vi "NML Data Acquisition Setup 1.00.vi"(9 "Parameters Input":T1={"Magnetic Field"=0.0, "Temperature"=0.0, "Exposure Time"=0.0, "Mag ID string"="", "User Name"="Albert Einstein", "Comments"="", "SaveComments?"=1, "X-Axis Unit"=1, "Delimiter"=0, "File Format"=0, "Sample Name"="Sample1"} {"File Format" items=["Macintosh (EOL: CR)", "Unix (EOL: LF)", "DOS/Windows (EOL: CR+LF)"]; "Delimiter" items=["TAB", "COMMA", "SPACE"]; "X-Axis Unit" items=["Point #", "nm", "eV", "meV", "cm-1"]; "SaveComments?" items=["Bare data only", "Saved in the Header Area", "Saved as a Parameter File"]; "Exposure Time" format="%.2f"; "Temperature" format="%.2f"; "Magnetic Field" format="%.2f"}) -> (0 "McP Scan Parameter":T2={"McP on?"=TRUE, "Wait"=0.0, "X-Axis Unit String"="", "Data Format"=0, "Scanning Pattern:"=0, "Spex on?"=TRUE} {"Scanning Pattern:" items=["Uniform Points ", "User Defined Point Pattern ", "Time-Drive"]; "Data Format" items=["Original", "1024rows X 2cloumns", "Future Use"]; "Wait" format="%.2f"}, 3 "Parameters Output":T1={"Magnetic Field"=0.0, "Temperature"=0.0, "Exposure Time"=0.0, "Mag ID string"="", "User Name"="Albert Einstein", "Comments"="", "SaveComments?"=1, "X-Axis Unit"=1, "Delimiter"=0, "File Format"=0, "Sample Name"="Sample1"} {"File Format" items=["Macintosh (EOL: CR)", "Unix (EOL: LF)", "DOS/Windows (EOL: CR+LF)"]; "Delimiter" items=["TAB", "COMMA", "SPACE"]; "X-Axis Unit" items=["Point #", "nm", "eV", "meV", "cm-1"]; "SaveComments?" items=["Bare data only", "Saved in the Header Area", "Saved as a Parameter File"]; "Exposure Time" format="%.2f"; "Temperature" format="%.2f"; "Magnetic Field" format="%.2f"})   [LabVIEW 2024]
doc: "VI which calls the appropriate GPIB routines for a variety of instruments.\nScott Hannahs, NHMFL-FSU, Nov. 1993"
uses:
  Sub Controls/NML GPIB List.ctl
  Sub VIs/McP Parameter.ctl
  xwei previous work/CCD Project/Subroutines/Parameters#1.ctl
  Globals and TypeDefs/Global Varibal Control.vi
panel:
  in  "Data Format":u8(ring)=1 items=["Original", "1024rows X 2cloumns", "Future Use"]
  in  "Spex1680 on?":bool=TRUE caption="Off"
  in  "X-Axis Unit String":string[](array[string])=["nm", "nm", "eV", "meV", "cm_1"]
  out "GPIB Status":string
  in  "ScanPattern":string="1.300000\r1.310000\r1.320000\r1.330000\r1.340000\r1.350000\r1.360000\r1.370000\r1.380000\r1.390000\r1.400000\r"
  in  "Logcluster":T3
  in  "Wait":dbl=1.0 caption="Wait(sec)" min=0.0 max=10000.0 format="%.1f"
  in  "Cancel":bool
  in  "Scanning Pattern:":u32(ring) items=["Uniform Points (Stop-&-Go)", "User Defined Point Pattern (Stop-&-Go)", "Time-Drive (Spectrometer moves at a constant speed)"]
  in  "End Point":dbl=1600.0 min=0.0 max=1000000.0 format="%.3f"
  in  "#Points":u16=100 min=2
  in  "Step":dbl=6.0 min=1e-05 format="%.3f"
  in  "Start Point":dbl=1000.0 min=0.0 max=1000000.0 format="%.3f"
  out "Clock":string="10:27:18 AM"
  in  "McP on?":bool=TRUE caption="Off"
  in  "Done?":bool
  in  "BusScan?":bool
  in  "SaveComments?":u16(ring)=1 items=["Bare data only", "Saved in the Header Area", "Saved as a Parameter File"]
  in  "Delimiter":u16(ring) items=["TAB", "COMMA", "SPACE"]
  in  "File Format":u16(ring) items=["Macintosh (EOL: CR)", "Unix (EOL: LF)", "DOS/Windows (EOL: CR+LF)"]
  in  "User Name":string="Conan The Scientist"
  in  "Sample Name":string="Sample1"
  in  "error in (no error)":errorcluster
  out "error out":errorcluster
  # "Scanning Panel"
  # "User Profile Panel"
  # "GPIB Instruments Panel"
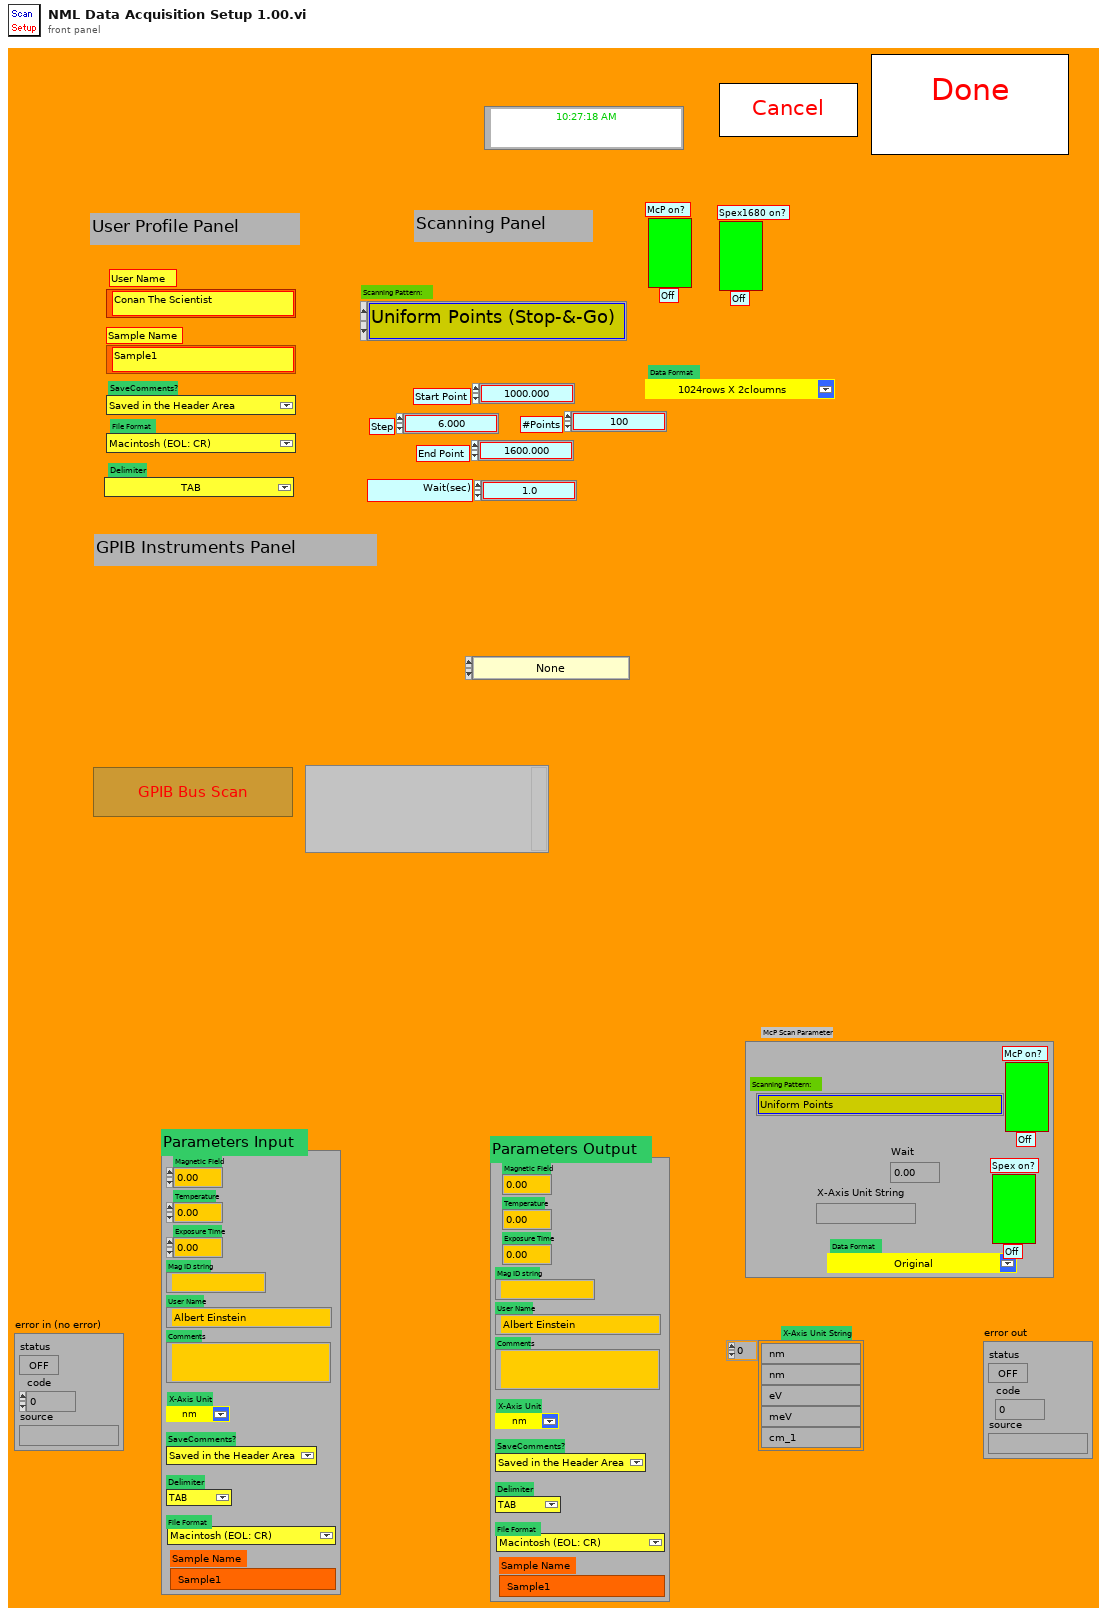
[diagram p1: front panel]
types:
  T1 = typedef "Parameters#1.ctl" = cluster{"Magnetic Field":dbl, "Temperature":dbl, "Exposure Time":dbl, "Mag ID string":string, "User Name":string, "Comments":string, "SaveComments?":u16, "X-Axis Unit":u16, "Delimiter":u16, "File Format":u16, "Sample Name":string}
  T2 = typedef "McP Parameter.ctl" = cluster{"McP on?":bool, "Wait":dbl, "X-Axis Unit String":string, "Data Format":u8, "Scanning Pattern:":u32, "Spex on?":bool}
  T3 = typedef "NML GPIB List.ctl" = enum16{"None", "Field", "Field - SCM1", "DMM", "DMM - HP 34401", "Keithley 2XXX", "Running DMM Ave", "Running HP34401", "Running K2XXX Ave", "SRS 830 - CH 1", "SRS 830 - CH1 & 2", "SRS PTC10", "Signal Rec 7265 - X", "Signal Rec 7265 - X&Y", "DRC 93C - Sample", "DRC 93C - Control", "DRC 93C - Sam&Con", "CryoCon Sensor A", "CryoCon Sensor B", "Cond 20C Sensor 1", "Cond 20C Sensor 2", "LS 336 Read", "LS 340 Read", "LS 370 Read", "LS 370 Select", "AVS 46 Bridge", "BLM Rotator Read Position", "Linear Research 700", "LR 700 Select", "Keithley 3330 - LCZ", "A-H Capacitance", "Digital Integrator", "SRS 400 Phot Ctr", "LakeShore VSM", "AMI He Level Meter", "Time Stamp", "Wait", "Invert Current", "K230 Linear V", "K230 VÅB^2", "Temp Ramp", "Power Ramp", "Freq Sweep", "LTC Stable T", "Scanner Step", "IMS Stepper Increment", "BLM Stepper Increment", "Omega CNi32"}
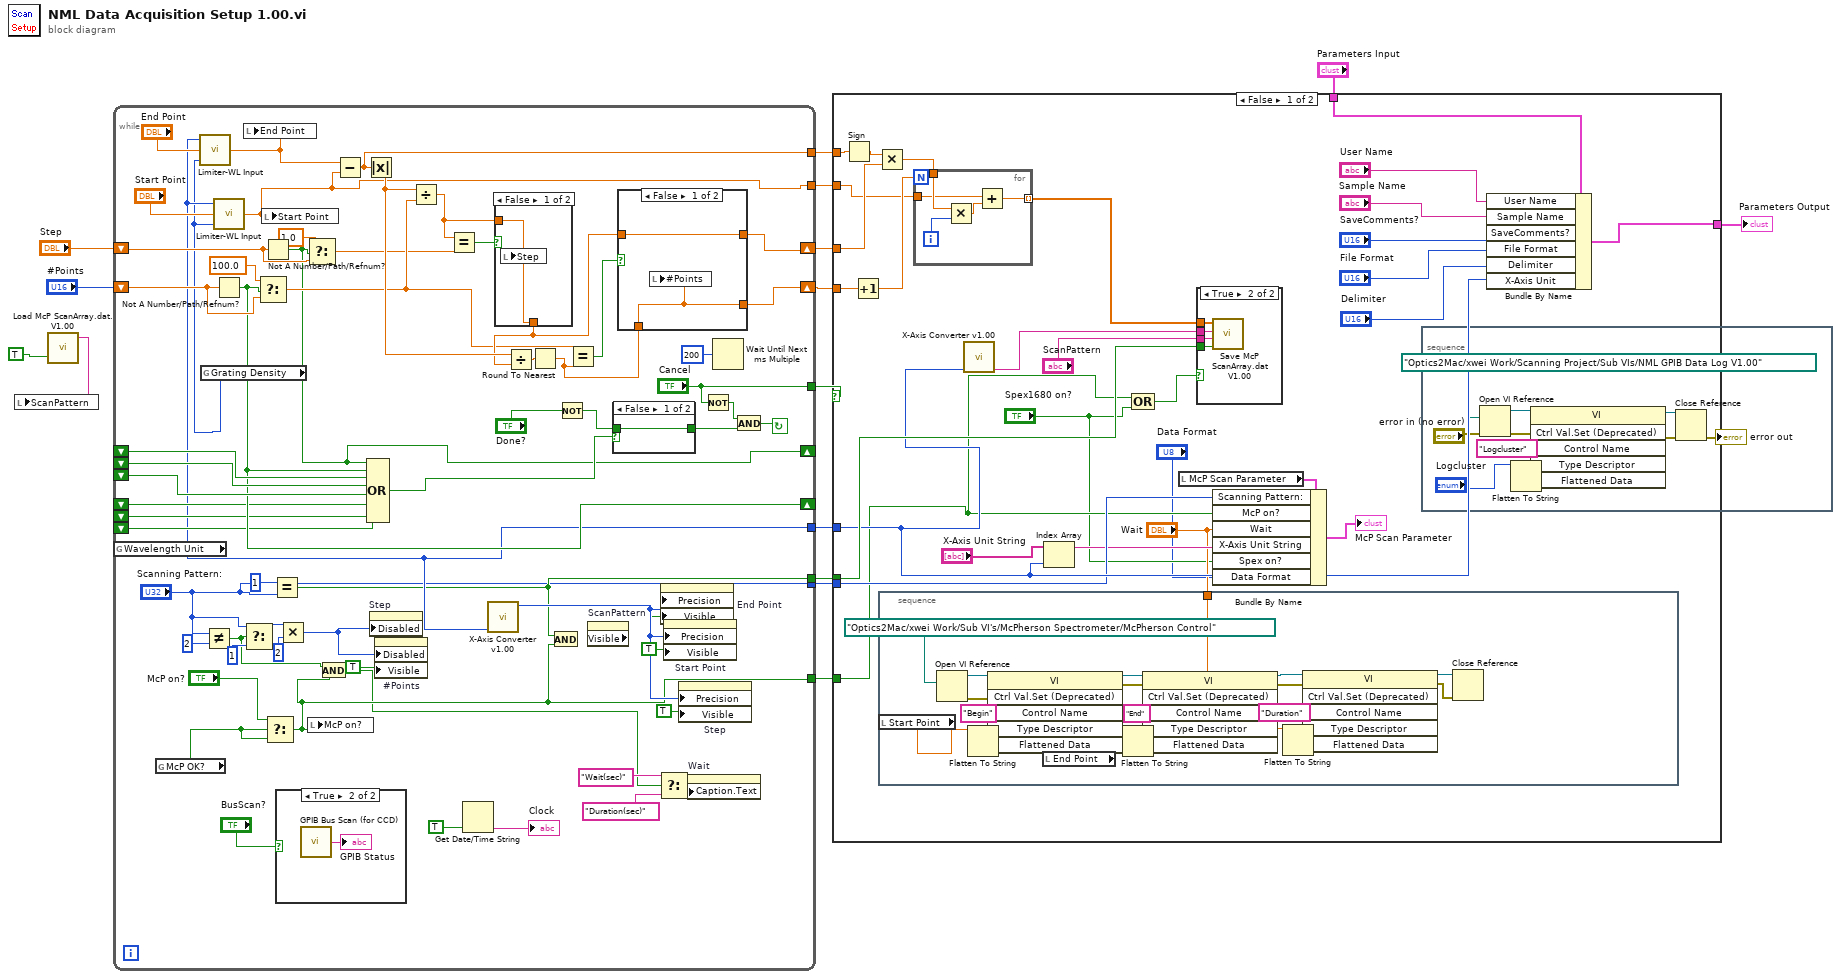
[diagram p0: block diagram]
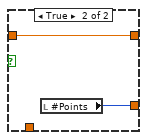
[diagram p4: hidden frame]
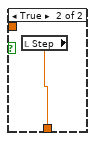
[diagram p5: hidden frame]
diagram:
  n1 = call "Load McP ScanArray.dat.V1.00.vi"("WholeArray?"=TRUE) -> ("ScanPattern"=w8:string)  [unwired: 1 in, 2 out]
  n2 = local write "ScanPattern"(w8) -> ()
  n3 = while {
    tunnel: ["Scanning Pattern:"] -> w1
    tunnel: [w20] -> w2
    tunnel: [w26] -> w5
    shift-left: _ -> [w45]
    shift-left: _ -> [w46]
    shift-left: _ -> [w47]
    shift-right: [w48] -> _
    shift-left: _ -> [w50]
    shift-left: _ -> [w51]
    shift-left: _ -> [w49]
    shift-right: [w52] -> _
    tunnel: [w64] -> w6
    tunnel: [w33] -> w7
    tunnel: [w65] -> w10
    tunnel: ["Cancel"] -> w12
    shift-left: "#Points" -> [w57]
    shift-right: [w67] -> w11
    shift-left: "Step" -> [w55]
    shift-right: [w69] -> w9
    stop <- w41 continue-if-true
    w18 = TRUE ("Write Attribute")
    n4 = global read "Global Varibal Control.vi" "Wavelength Unit"() -> (w33:u8)
    n5 = global read "Global Varibal Control.vi" "McP OK?"() -> (w32:bool)
    n6 = global read "Global Varibal Control.vi" "Grating Density"() -> (w22:u8)
    n7 = call "Limiter-WL Input.vi"("Current Grating Density"=w22, "Central WL Input"="End Point", "X-Axis"=w33) -> ("Central WL output"=w62:dbl)
    n8 = Not Equal?(x="Scanning Pattern:", y=u32 2) -> (x != y?=w28:bool)
    n9 = call "Limiter-WL Input.vi"("Current Grating Density"=w22, "Central WL Input"="Start Point", "X-Axis"=w33) -> ("Central WL output"=w64:dbl)
    n10 = Not A Number/Path/Refnum?(number/path/refnum=w57) -> (NaN/Path/Refnum?=w48:bool)
    n11 = local write "End Point"(w62) -> ()
    n12 = Select(t="Scanning Pattern:", s=w28, f=u32 1 ("t")) -> (s? t:f=w30:u32)
    n13 = Select(t=100.0 ("f"), s=w48, f=w57) -> (s? t:f=w60:dbl)
    n14 = local write "Start Point"(w64) -> ()
    n15 = Not A Number/Path/Refnum?(number/path/refnum=w55) -> (NaN/Path/Refnum?=w52:bool)
    n16 = Select(t="McP on?", s=w32, f=w32) -> (s? t:f=w20:bool)
    n17 = Equal?(x=u32 1, y="Scanning Pattern:") -> (x = y?=w26:bool)
    n18 = case shown="True" "BusScan?" {
      frame False {
      }
      frame True {
        n19 = call "GPIB Bus Scan (for CCD).vi"() -> (0:→"GPIB Status":string)  [unwired: 1 in]
      }
    }
    n20 = Multiply(x=w30, y=u32 2) -> (x*y=w39:u32)
    n21 = Select(t=1.0 ("f"), s=w52, f=w55) -> (s? t:f=w59:dbl)
    n22 = local write "McP on?"(w20) -> ()
    n23 = And(x=w28, y=w20) -> (x .and. y?=w16:bool)
    n24 = Subtract(x=w62, y=w64) -> (x-y=w65:dbl)
    n25 = Absolute Value(x=w65) -> (abs(x)=w72:dbl)
    n26 = Compound Arithmetic op=OR(w52, w48, w49, w51, w50, w47, w46, w45) -> (w54:bool)
    n27 = property on="Step" class="DigNum (strict)"("Disabled"=w39) -> ()  [unwired: 2 in, 2 out]
    n28 = property on="#Points" class="DigNum (strict)"("Disabled"=w39, "Visible"=TRUE ("Write Attribute")) -> ()  [unwired: 2 in, 2 out]
    n29 = Divide(x=w72, y=w60) -> (x/y=w73:dbl)
    n30 = Equal?(x=w73, y=w59) -> (x = y?=w74:bool)
    n31 = Get Date/Time String(want seconds? (F)=TRUE) -> (time string=→"Clock":string)  [unwired: 2 in, 1 out]
    n32 = call "X-Axis Converter v1.00.vi"("X-Axis Unit"=w33) -> ("Precision"=w38:i32)  [unwired: 4 in, 3 out]
    n33 = case shown="False" w74 {
      tunnel: w73 -> [w84 _]
      tunnel: [w84 w85] -> w68
      frame False {
        n34 = local write "Step"(w84) -> ()
      }
      frame True {
        n35 = local read "Step"() -> (w85:dbl)
      }
    }
    n36 = Divide(x=w72, y=w68) -> (x/y=w75:dbl)
    n37 = Round To Nearest(number=w75) -> (nearest integer value=w70:dbl)
    n38 = And(x=w26, y=w20) -> ()  [unwired: 1 out]
    n39 = Not(x="Done?") -> (.not. x?=w53:bool)
    n40 = Equal?(x=w60, y=w70) -> (x = y?=w71:bool)
    n41 = property on="ScanPattern" class="Str" props=["Visible"]() -> ()  [unwired: 2 in, 3 out]
    n42 = case shown="False" w54 {
      selector: w54 -> [_ w79]
      tunnel: [w78 w79] -> w42
      tunnel: w53 -> [w78 _]
      frame False {
      }
      frame True {
      }
    }
    n43 = case shown="False" w71 {
      tunnel: w70 -> [w80 _]
      tunnel: w68 -> [w81 w82]
      tunnel: [w81 w82] -> w69
      tunnel: [w80 w83] -> w67
      frame False {
        n44 = local write "#Points"(w80) -> ()
      }
      frame True {
        n45 = local read "#Points"() -> (w83:u16)
      }
    }
    n46 = Select(t="Wait(sec)", s=w16, f="Duration(sec)") -> (s? t:f=w23:string)
    n47 = property on="End Point" class="DigNum (strict)"("Precision"=w38, "Visible"=w18) -> ()  [unwired: 2 in, 2 out]
    n48 = property on="Start Point" class="DigNum (strict)"("Precision"=w38, "Visible"=w18) -> ()  [unwired: 2 in, 2 out]
    n49 = property on="Step" class="DigNum (strict)"("Precision"=w38, "Visible"=TRUE ("Write Attribute")) -> ()  [unwired: 2 in, 2 out]
    n50 = property on="Wait" class="DigNum (strict)"("Caption.Text"=w23) -> ()  [unwired: 2 in, 2 out]
    n51 = Not(x="Cancel") -> (.not. x?=w43:bool)
    n52 = Wait Until Next ms Multiple(millisecond multiple=u32 200) -> ()  [unwired: 1 out]
    n53 = And(x=w43, y=w42) -> (x .and. y?=w41:bool)
  }
  n54 = case shown="False" w12 {
    tunnel: w11 -> [w105 _]
    tunnel: w10 -> [w109 _]
    tunnel: w9 -> [w107 _]
    tunnel: w7 -> [w93 _]
    tunnel: w6 -> [w103 _]
    tunnel: w5 -> [w102 _]
    tunnel: [w100 w156] -> w3
    tunnel: "Parameters Input" -> [w101 w156]
    tunnel: w2 -> [w89 _]
    tunnel: w1 -> [w92 _]
    frame False {
      n55 = Sign(1:w109) -> (0:w108:dbl)
      n56 = Increment(x=w105) -> (x+1=w104:dbl)
      n57 = Multiply(x=w108, y=w107) -> (x*y=w106:dbl)
      n58 = stacked-sequence {
        tunnel: "Wait" -> [w116]
        frame #0 {
          n59 = local read "Start Point"() -> (w129:dbl)
          n60 = Open VI Reference(vi path=path "/Optics2Mac/xwei Work/Sub VI's/McPherson Spectrometer/McPherson Control") -> (vi reference=w134:refnum<vi>, error out=w130:errorcluster)  [unwired: 5 in]
          n61 = Flatten To String(anything=w129) -> (data string=w131:string, type string=w132:i16[])  [unwired: 3 in, 1 out]
          n62 = invoke class="VI" method="Ctrl Val.Set (Deprecated)"(reference=w134, error in=w130, "Control Name"="Begin", "Type Descriptor"=w132, "Flattened Data"=w131) -> (reference out=w122:refnum<vi>, error out=w121:errorcluster)  [unwired: 1 in, 4 out]
          n63 = local read "End Point"() -> (w115:dbl)
          n64 = Flatten To String(anything=w115) -> (data string=w126:string, type string=w127:i16[])  [unwired: 3 in, 1 out]
          n65 = invoke class="VI" method="Ctrl Val.Set (Deprecated)"(reference=w122, error in=w121, "Control Name"="End", "Type Descriptor"=w127, "Flattened Data"=w126) -> (reference out=w119:refnum<vi>, error out=w120:errorcluster)  [unwired: 1 in, 4 out]
          n66 = Flatten To String(anything=w116) -> (data string=w123:string, type string=w124:i16[])  [unwired: 3 in, 1 out]
          n67 = invoke class="VI" method="Ctrl Val.Set (Deprecated)"(reference=w119, error in=w120, "Control Name"="Duration", "Type Descriptor"=w124, "Flattened Data"=w123) -> (reference out=w118:refnum<vi>, error out=w117:errorcluster)  [unwired: 1 in, 4 out]
          n68 = Close Reference(reference=w118, error in (no error)=w117) -> ()  [unwired: 1 out]
        }
      }
      n69 = for {
        N: w104 -> [_]
        tunnel: w106 -> [w154]
        tunnel: [w152] -> w114 mode=indexing
        tunnel: w103 -> [w151]
        i -> [w155]
        n70 = Multiply(x=w154, y=w155) -> (x*y=w153:dbl)
        n71 = Add(x=w151, y=w153) -> (x+y=w152:dbl)
      }
      n72 = call "X-Axis Converter v1.00.vi"("X-Axis Unit"=w93) -> ("UnitFormatString"=w110:string)  [unwired: 4 in, 3 out]
      n73 = Index Array(array="X-Axis Unit String", index=w93) -> (element=w91:string)
      n74 = Compound Arithmetic op=OR(w89, "Spex1680 on?") -> (w88:bool)
      n75 = local read "McP Scan Parameter"() -> (w112:T2)
      n76 = case shown="True" w88 {
        tunnel: w114 -> [_ w139]
        tunnel: "ScanPattern" -> [_ w138]
        tunnel: w110 -> [_ w137]
        tunnel: w102 -> [_ w136]
        frame False {
        }
        frame True {
          n77 = call "Save McP ScanArray.dat V1.00.vi"("ScanPattern?"=w136, "ScanPattern"=w138, "format (%.3f)"=w137, "1D data"=w139) -> ()  [unwired: 3 in]
        }
      }
      n78 = Bundle By Name(cluster=w112, "Scanning Pattern:"=w92, "McP on?"=w89, "Wait"="Wait", "X-Axis Unit String"=w91, "Spex on?"="Spex1680 on?", "Data Format"="Data Format") -> (→"McP Scan Parameter":T2)
      n79 = stacked-sequence {
        frame #0 {
          n80 = Open VI Reference(vi path=path "/Optics2Mac/xwei Work/Scanning Project/Sub VIs/NML GPIB Data Log V1.00", error in (no error)="error in (no error)") -> (vi reference=w149:refnum<vi>, error out=w143:errorcluster)  [unwired: 4 in]
          n81 = Flatten To String(anything="Logcluster") -> (data string=w146:string, type string=w147:i16[])  [unwired: 3 in, 1 out]
          n82 = invoke class="VI" method="Ctrl Val.Set (Deprecated)"(reference=w149, error in=w143, "Control Name"="Logcluster", "Type Descriptor"=w147, "Flattened Data"=w146) -> (reference out=w142:refnum<vi>, error out=w141:errorcluster)  [unwired: 1 in, 4 out]
          n83 = Close Reference(reference=w142, error in (no error)=w141) -> (error out=→"error out":errorcluster)
        }
      }
      n84 = Bundle By Name(cluster=w101, "User Name"="User Name", "Sample Name"="Sample Name", "SaveComments?"="SaveComments?", "File Format"="File Format", "Delimiter"="Delimiter", "X-Axis Unit"=w93) -> (w100:T1)
    }
    frame True {
    }
  }
  "Parameters Output" <- w3
